vi "getCSVtoken.vi"(11 "packet string":string) -> (3 "remainder of packet":string, 4 "token":i32)   [LabVIEW 2012]
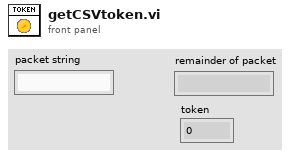
[diagram p1: front panel]
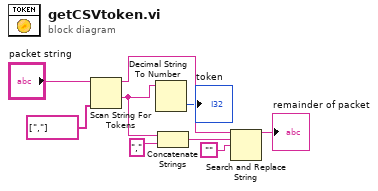
[diagram p0: block diagram]
diagram:
  n1 = Scan String For Tokens(6:string[] [","] ("delimiters (\\s,\\t,\\r,\\n)"), 9:"packet string") -> (1:w2:string, 3:w7:string)  [unwired: 4 in, 2 out]
  n2 = Decimal String To Number(string=w2) -> (number=→"token":i32)  [unwired: 2 in, 1 out]
  n3 = Concatenate Strings(w2, "," ("string")) -> (w3:string)
  n4 = Search and Replace String(input string=w7, search string=w3, replace string="") -> (result string=→"remainder of packet":string)  [unwired: 5 in, 3 out]
